vi "LogForTriggerNext.vi"(8 "error in (no error)":errorcluster, 10 "Log":string) -> (0 "error out":errorcluster)   [LabVIEW 2020]
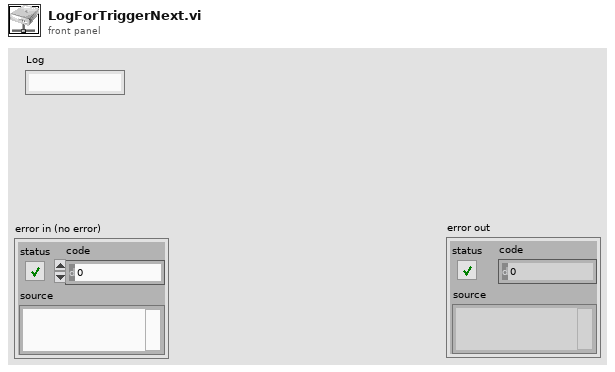
[diagram p1: front panel]
types:
  T1 = enum16{"open", "replace", "create", "open or create", "replace or create", "replace or create with confirmation"}
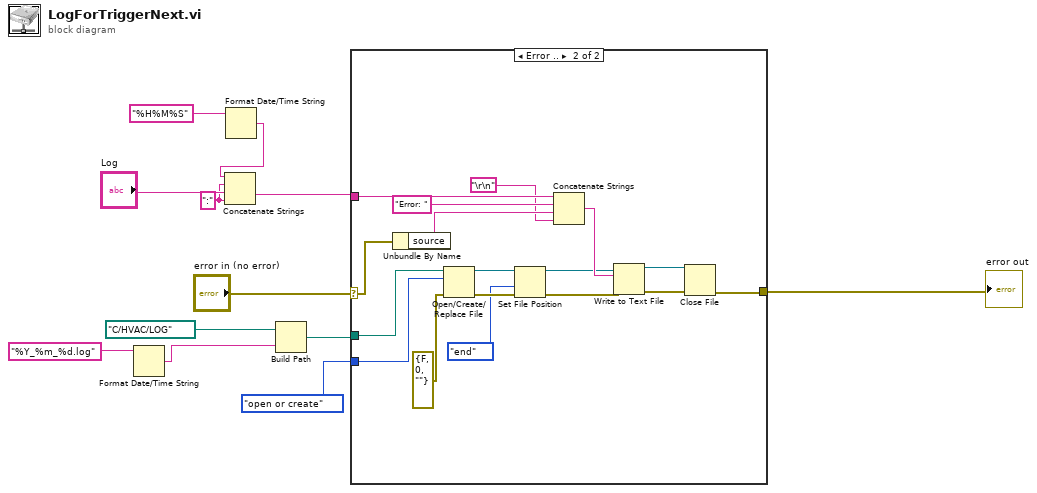
[diagram p0: block diagram]
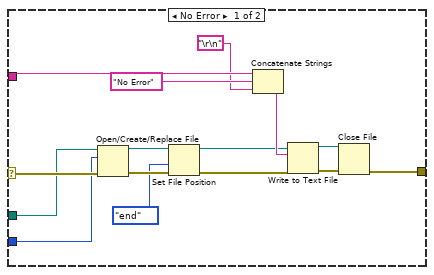
[diagram p2: hidden frame]
diagram:
  w2 = ":" ("string")
  n1 = Format Date/Time String(time format string (%c)="%Y_%m_%d.log") -> (date/time string=w6:string)  [unwired: 2 in]
  n2 = Format Date/Time String(time format string (%c)="%H%M%S") -> (date/time string=w1:string)  [unwired: 2 in]
  n3 = Concatenate Strings(w1, w2, "Log", w2) -> (w4:string)
  n4 = Build Path(base path=path "C:/HVAC/LOG" ("file path (use dialog)"), name or relative path=w6) -> (appended path=w9:path)
  n5 = case shown="Error .." "error in (no error)" {
    selector: "error in (no error)" -> [w27 w35]
    tunnel: [w24 w42] -> w11
    tunnel: T1."open or create" ("operation (0:open)") -> [w23 w40]
    tunnel: w9 -> [w22 w39]
    tunnel: w4 -> [w21 w38]
    frame No Error {
      n6 = Open/Create/Replace File(file path (use dialog)=w22, error in=w27, operation (0:open)=w23) -> (refnum out=w16:refnum<file>, error out=w17:errorcluster)  [unwired: 3 in, 1 out]
      n7 = Set File Position(refnum=w16, from (0:start)=enum16{"start", "end", "current"}."end", error in=w17) -> (refnum out=w15:refnum<file>, error out=w14:errorcluster)  [unwired: 1 in]
      n8 = Concatenate Strings(w21, "No Error" ("string"), "\r\n") -> (w19:string)
      n9 = Write to Text File(file (use dialog)=w15, text=w19, error in=w14) -> (refnum out=w25:refnum<file>, error out=w26:errorcluster)  [unwired: 1 in, 1 out]
      n10 = Close File(refnum=w25, error in=w26) -> (error out=w24:errorcluster)  [unwired: 1 out]
    }
    frame Error {
      n11 = Unbundle By Name(w35) -> ("source"=w34:string)
      n12 = Open/Create/Replace File(file path (use dialog)=w39, error in=errorcluster {"status"=FALSE, "code"=0, "source"=""}, operation (0:open)=w40) -> (refnum out=w31:refnum<file>, error out=w32:errorcluster)  [unwired: 3 in, 1 out]
      n13 = Set File Position(refnum=w31, from (0:start)=enum16{"start", "end", "current"}."end", error in=w32) -> (refnum out=w30:refnum<file>, error out=w29:errorcluster)  [unwired: 1 in]
      n14 = Concatenate Strings(w38, "Error: " ("string"), w34, "\r\n") -> (w36:string)
      n15 = Write to Text File(file (use dialog)=w30, text=w36, error in=w29) -> (refnum out=w43:refnum<file>, error out=w44:errorcluster)  [unwired: 1 in, 1 out]
      n16 = Close File(refnum=w43, error in=w44) -> (error out=w42:errorcluster)  [unwired: 1 out]
    }
  }
  "error out" <- w11
